vi "Load SLSC Switch Module Configuration.vi"(8 "error in":errorcluster, 9 "product name":string, 10 "switches json file":path, 11 "slsc switch custom device in":T1 format="%.0x") -> (0 "error out":errorcluster, 3 "slsc switch custom device out":T1 format="%.0x")   [LabVIEW 2020, in "SLSC Switch Scripting.lvlib"]
doc: "Configures the SLSC Switch custom device using the switches JSON file. The contents of this JSON file are stored on the SLSC module or provided separately by the module vendor."
uses:
  SLSC Switch Scripting.lvlib
  <vilib>/NI VeriStand/Custom Device API/Custom Device Item Ref.ctl
  <vilib>/NI VeriStand/Custom Device API/Custom Device API.lvlib
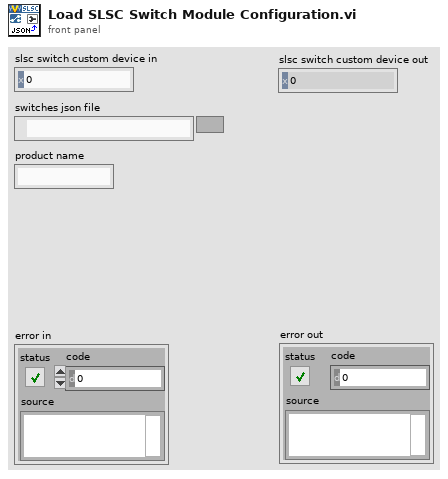
[diagram p1: front panel]
types:
  T1 = typedef "Custom Device API.lvlib/Custom Device Item Ref.ctl" = u64
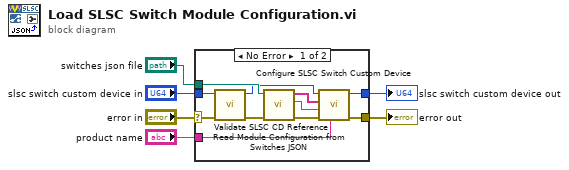
[diagram p0: block diagram]
diagram:
  n1 = case shown="No Error" "error in" {
    selector: "error in" -> [w8 w18]
    tunnel: "slsc switch custom device in" -> [w10 w19]
    tunnel: [w15 w18] -> w3
    tunnel: [w16 w19] -> w4
    tunnel: "switches json file" -> [w14 _]
    tunnel: "product name" -> [w13 _]
    frame No Error {
      n2 = call "Validate SLSC CD Reference.vi"("error in"=w8, "slsc switch custom device in"=w10) -> ("error out"=w7:errorcluster, "slsc switch custom device out"=w9:T1)  [unwired: 8 in]
      n3 = call "Read Module Configuration from Switches JSON.vi"("error in"=w7, "switches json file"=w14) -> ("error out"=w17:errorcluster, "switches json"=w11:string, "topologies"=w12:string[])  [unwired: 7 in]
      n4 = call "Configure SLSC Switch Custom Device.vi"("product name"=w13, "error in"=w17, "switches json"=w11, "topologies"=w12, "slsc switch custom device in"=w9) -> ("error out"=w15:errorcluster, "slsc switch custom device out"=w16:T1)  [unwired: 5 in]
    }
    frame Error {
    }
  }
  "error out" <- w3
  "slsc switch custom device out" <- w4
